vi "Calculate-Cycle time (Eqn).vi"(9 "[ROI Time (us)]":dbl[](array[numeric]), 11 "Header data":T1={"Number of POI"=0, "Number of Miniscans"=0, "Number of Trials"=0, "Number of Cycles "=0, "# Averaged Frames"=0, "Laser power (%)"=0, "Pockels"=0.0, "Acquisition Length (sec)"=0.0, "Fill time (us)"=0.0, "DwellTime (us)"=0.0, "Miniscan Dwell time per pixel (us)"=0.0, "PMT 1"=0.0, "PMT 2"=0.0, "Back Apperture"=0.0, "Zoom"=0.0, "Number of Pixels in Miniscan"=0, "Frame Size"=200, "Field of View"=0.0, "X centre"=0.0, "Y centre"=0.0, "AOL Z"=0.0} {"Frame Size" items=["100X100"=100, "128X128"=128, "200X200"=200, "256X256"=256, "512X512"=512, "1024x1024"=1024, "2048x2048"=2048]; "Back Apperture" format="%#.6g"; "Pockels" format="%#.6g"; "PMT 2" format="%#.6g"; "PMT 1" format="%#.6g"; "Miniscan Dwell time per pixel (us)" format="%#.6g"; "Zoom" format="%#.6g"; "DwellTime (us)" format="%#.6g"; "Acquisition Length (sec)" format="%#.6g"; "Fill time (us)" format="%#.6g"}) -> (3 "Cycle Time (us)":dbl)   [LabVIEW 2020]
uses:
  Experiment header interface/Typedefs/Header parameters cluster-Zstack.ctl
  Typedefs/Frame Size.ctl
panel:
  # "Zstack header parameters"
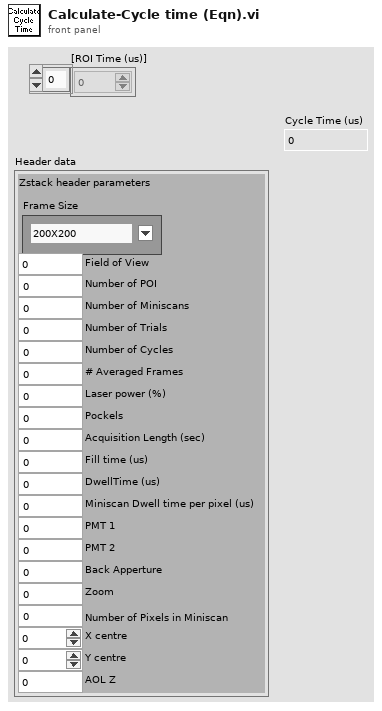
[diagram p1: front panel]
types:
  T1 = typedef "Header parameters cluster-Zstack.ctl" = cluster{"Number of POI":u16, "Number of Miniscans":u16, "Number of Trials":u16, "Number of Cycles ":u16, "# Averaged Frames":u16, "Laser power (%)":u8, "Pockels":dbl, "Acquisition Length (sec)":dbl, "Fill time (us)":dbl, "DwellTime (us)":dbl, "Miniscan Dwell time per pixel (us)":dbl, "PMT 1":dbl, "PMT 2":dbl, "Back Apperture":dbl, "Zoom":dbl, "Number of Pixels in Miniscan":u16, "Frame Size":T2, "Field of View":dbl, "X centre":dbl, "Y centre":dbl, "AOL Z":dbl}
  T2 = typedef "Frame Size.ctl" = u16
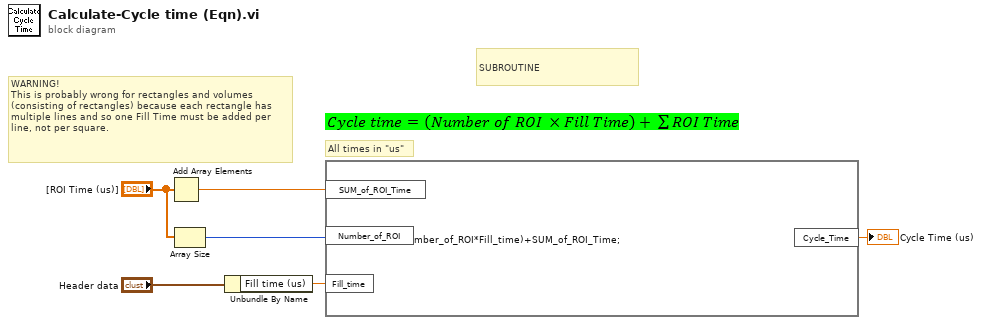
[diagram p0: block diagram]
diagram:
  # "WARNING!\nThis is probably wrong for rectangles and volumes (consisting of rectangles) because each rectangle has multiple lines and so one Fill Time must be added per line, not per square."
  # "SUBROUTINE"
  # "All times in \"us\""
  n1 = Add Array Elements(numeric array="[ROI Time (us)]") -> (sum=w1:dbl)
  n2 = Array Size(array="[ROI Time (us)]") -> (size(s)=w3:i32)
  n3 = Unbundle By Name("Header data") -> ("Fill time (us)"=w5:dbl)
  n4 = formula code="Cycle_Time=(Number_of_ROI*Fill_time)+SUM_of_ROI_Time;"("SUM_of_ROI_Time"=w1, "Number_of_ROI"=w3, "Fill_time"=w5) -> ("Cycle_Time"=→"Cycle Time (us)":dbl)
